vi "GetDataFlowProcess.vi"(8 "error in (no error)":errorcluster, 10 "type":T1, 11 "source":string) -> (0 "error out":errorcluster, 1 "found":bool, 2 "last block":bool, 3 "Dataflow process":string)   [LabVIEW 2017, in "DataFlow.lvlib"]
uses:
  <vilib>/addons/InsightCM/Devices/Shared/Common/DataFlow/DataFlow.lvlib
  <vilib>/addons/InsightCM/Devices/Shared/Common/DataFlow/controls/Type.ctl
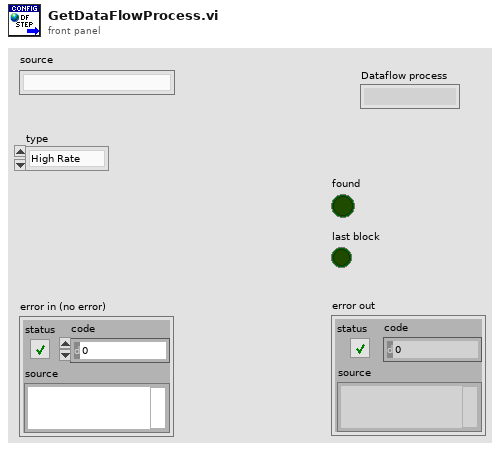
[diagram p1: front panel]
types:
  T1 = typedef "DataFlow.lvlib/Type.ctl" = enum16{"High Rate", "Low Rate", "Burst Mode"}
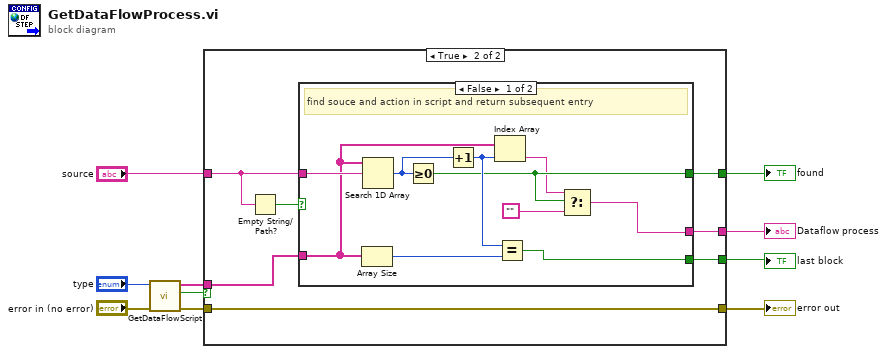
[diagram p0: block diagram]
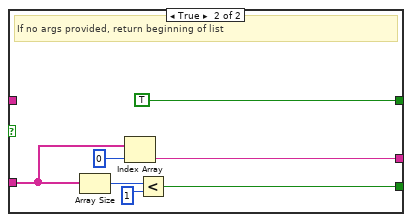
[diagram p3: hidden frame]
diagram:
  n1 = call <vilib>:"GetDataFlowScript.vi"("error in (no error)"="error in (no error)", "type"="type") -> ("error out"=w4:errorcluster, "found"=w2:bool, "Dataflow script"=w3:string[])  [unwired: 7 in]
  n2 = case shown="True" w2 {
    selector: w2 -> [w12 _]
    tunnel: [w11 w14] -> w10
    tunnel: [w12 w18] -> w9
    tunnel: w4 -> [w11 w14]
    tunnel: "source" -> [_ w16]
    tunnel: [_ w19] -> w7
    tunnel: [_ w17] -> w6
    tunnel: w3 -> [_ w13]
    frame False {
    }
    frame True {
      n3 = Empty String/Path?(string/path=w16) -> (empty?=w15:bool)
      n4 = case shown="False" w15 {
        tunnel: w16 -> [w29 _]
        tunnel: [w20 w35] -> w19
        tunnel: [w23 TRUE] -> w18
        tunnel: w13 -> [w26 w34]
        tunnel: [w28 w31] -> w17
        frame False {
          # "find souce and action in script and return subsequent entry"
          n5 = Array Size(array=w26) -> (size(s)=w25:i32)
          n6 = Search 1D Array(1D array=w26, element=w29) -> (index of element=w27:i32)  [unwired: 1 in]
          n7 = Greater Or Equal To 0?(x=w27) -> (x >= 0?=w23:bool)
          n8 = Increment(x=w27) -> (x+1=w24:i32)
          n9 = Index Array(array=w26, index=w24) -> (element=w21:string)
          n10 = Equal?(x=w24, y=w25) -> (x = y?=w28:bool)
          n11 = Select(t=w21, s=w23, f="") -> (s? t:f=w20:string)
        }
        frame True {
          # "If no args provided, return beginning of list"
          n12 = Array Size(array=w34) -> (size(s)=w33:i32)
          n13 = Index Array(array=w34, index=0) -> (element=w35:string)
          n14 = Less?(x=w33, y=1) -> (x < y?=w31:bool)
        }
      }
    }
  }
  "error out" <- w10
  "found" <- w9
  "Dataflow process" <- w7
  "last block" <- w6
